vi "Flush Error Queue.vi"(8 "error in (no error)":errorcluster, 11 "SOL-Server in":refnum<class "SOL-Server.lvclass">) -> (0 "error out":errorcluster, 2 "Errors":T1[](array[typedef]), 3 "SOL-Server out":refnum<class "SOL-Server.lvclass">)   [LabVIEW 2020, in "Summer of LabVIEW.lvlib" / "SOL-Server.lvclass"]
uses:
  SOL-Server.lvclass
  SOL-Server.lvclass/SOL-Server.ctl
  Error Log.ctl
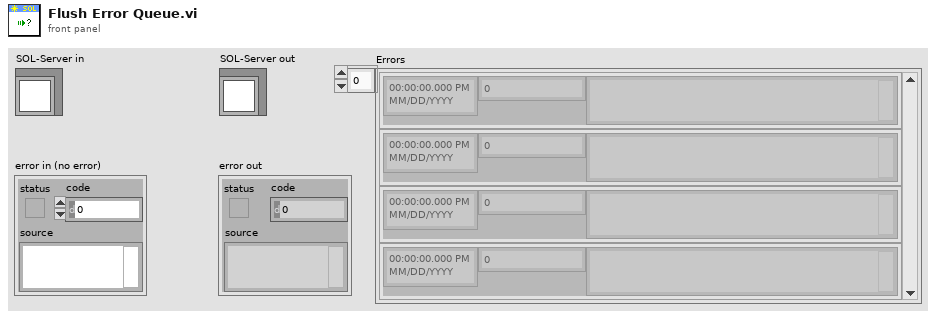
[diagram p1: front panel]
types:
  T1 = typedef "Summer of LabVIEW.lvlib/SOL-Server.lvclass/Error Log.ctl" = cluster{"Time Stamp":timestamp, "Code":i32, "Source":string}
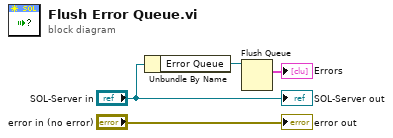
[diagram p0: block diagram]
diagram:
  n1 = Unbundle By Name("SOL-Server in") -> ("Error Queue"=w2:refnum<queue>)
  n2 = Flush Queue(queue=w2) -> (remaining elements=→"Errors":T1[])  [unwired: 1 in, 2 out]
  "error out" <- "error in (no error)"
  "SOL-Server out" <- "SOL-Server in"
